vi "Register Events to Source.vi"(8 "error in (no error)":errorcluster, 11 "Event Sink in":refnum<class "Event Sink.lvclass">) -> (0 "error out":errorcluster, 3 "Event Sink out":refnum<class "Event Sink.lvclass">)   [LabVIEW 2016, in "Event Source.lvlib" / "Event Sink.lvclass"]
doc: "This dinamic dispatch methods has to be overriddent by the child sink classes to register events to the source"
uses:
  Event Sink.lvclass
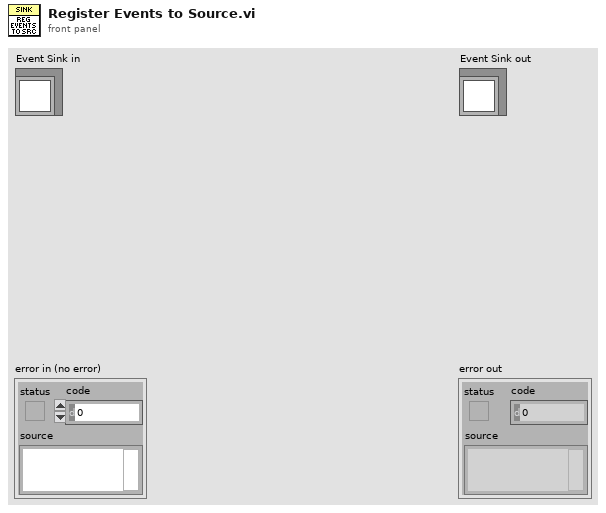
[diagram p1: front panel]
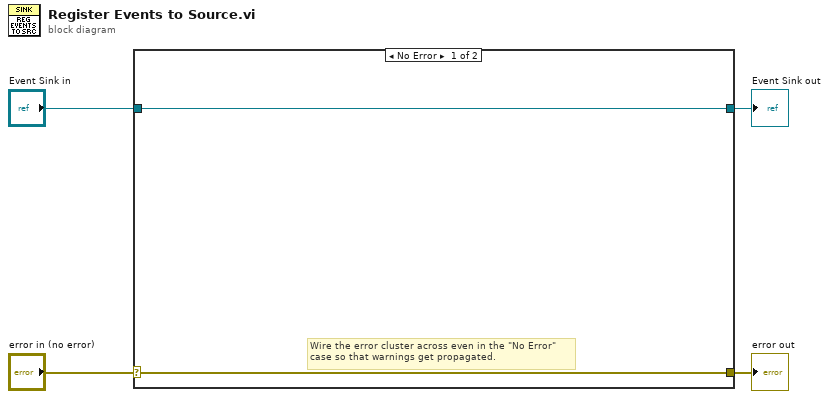
[diagram p0: block diagram]
diagram:
  n1 = case shown="No Error" "error in (no error)" {
    selector: "error in (no error)" -> [w5 w8]
    tunnel: [w5 w8] -> w3
    tunnel: [w6 w7] -> w1
    tunnel: "Event Sink in" -> [w6 w7]
    frame No Error {
      # "Wire the error cluster across even in the \"No Error\"\ncase so that warnings get propagated."
    }
    frame Error {
    }
  }
  "error out" <- w3
  "Event Sink out" <- w1
